vi "Function.vi"(8 "error in (no error)":errorcluster, 9 "Numeric B":T1, 10 "Numeric A":T1, 11 "Class in":refnum<class "Divide_EXT.lvclass">) -> (0 "error out":errorcluster, 2 "Result":T1, 3 "Class out":refnum<class "Divide_EXT.lvclass">)   [LabVIEW 2021, in "Divide_EXT.lvclass"]
uses:
  Divide_EXT.lvclass
  Type.ctl
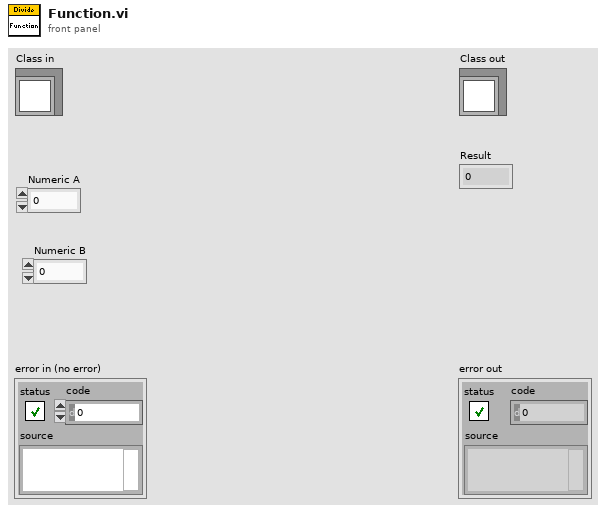
[diagram p1: front panel]
types:
  T1 = typedef "Divide_EXT.lvclass/Type.ctl" = ext
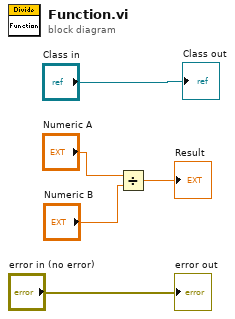
[diagram p0: block diagram]
diagram:
  n1 = Divide(x="Numeric A", y="Numeric B") -> (x/y=→"Result":T1)
  "error out" <- "error in (no error)"
  "Class out" <- "Class in"
